vi "Test_Window.vi"() -> ()   [LabVIEW 2018]
uses:
  _TypeDefs/Flags/Z900_navX_Flags_HardwareRevTypeDef.ctl
  _TypeDefs/Flags/Z900_navX_Flags_OmnimountConfigTypeDef.ctl
  _TypeDefs/Flags/Z900_navX_Flags_OpStatusTypeDef.ctl
  _TypeDefs/Flags/Z900_navX_Flags_CalibrationStatusTypeDef.ctl
  _TypeDefs/Z900_navX_SerialStreamTypeDef.ctl
  _TypeDefs/FRIC_navX_DeviceNumbersTypeDef.ctl
panel:
  in  "Tab Control":enum32{"Device 0", "Device 1"}(tab)
  out "Warning":bool
  in  "Change Serial Stream":bool
  out "Connected":bool
  out "Displacement":T1 {"Velocity X" format="%.8f"; "Velocity Y" format="%.8f"; "Velocity Z" format="%.8f"; "Displace X" format="%.8f"; "Displace Y" format="%.8f"; "Displace Z" format="%.8f"}
  out "MPUTemp":dbl format="%.2f"
  out "Board Information":T4 {"Board"."Hardware Revision" items=["navX-MXP"=33, "navX-Micro"=40]; "Omnimount Config" items=["DEFAULT", "X_UP", "X_DOWN", "Y_UP", "Y_DOWN", "Z_UP", "Z_DOWN"]}
  out "Linear Acceleration":cluster{"X":dbl, "Y":dbl, "Z":dbl} {"X" format="%.6f"; "Y" format="%.6f"; "Z" format="%.6f"}
  out "Quaternion":T5 {"Quat W" format="%.8f"; "Quat X" format="%.8f"; "Quat Y" format="%.8f"; "Quat Z" format="%.8f"}
  out "Status":T8 {"OP Status" items=["INITIALIZING", "SELFTEST_IN_PROGRESS", "ERROR", "IMU_AUTOCAL_IN_PROGRESS", "NORMAL"]; "Calibration Status" items=["IMU_CAL_STATE_MASK"=3, "IMU_CAL_STATE_INPROGRESS"=0, "IMU_CAL_STATE_ACCUMULATE"=1, "IMU_CAL_STATE_COMPLETE"=2]}
  out "YRPHfH":T9 {"Yaw" format="%.2f"; "Roll" format="%.2f"; "Pitch" format="%.2f"; "Heading" format="%.2f"; "Fused Heading" format="%.2f"}
  out "Timestamp":u32
  out "Error":bool
  out "error":errorcluster
  in  "Zero Yaw":bool
  in  "Zero Displacement":bool
  in  "Zero Velocity":bool
  out "Raw Values":T10 {"Accel X" format="%.8f"; "Accel Y" format="%.8f"; "Accel Z" format="%.8f"; "Gyro X" format="%.8f"; "Gyro Y" format="%.8f"; "Gyro Z" format="%.8f"; "Mag X" format="%.8f"; "Mag Y" format="%.8f"; "Mag Z" format="%.8f"}
  in  "Stream Type":T11=enum."AHRSAndPositioning"
  in  "Device Number":T12
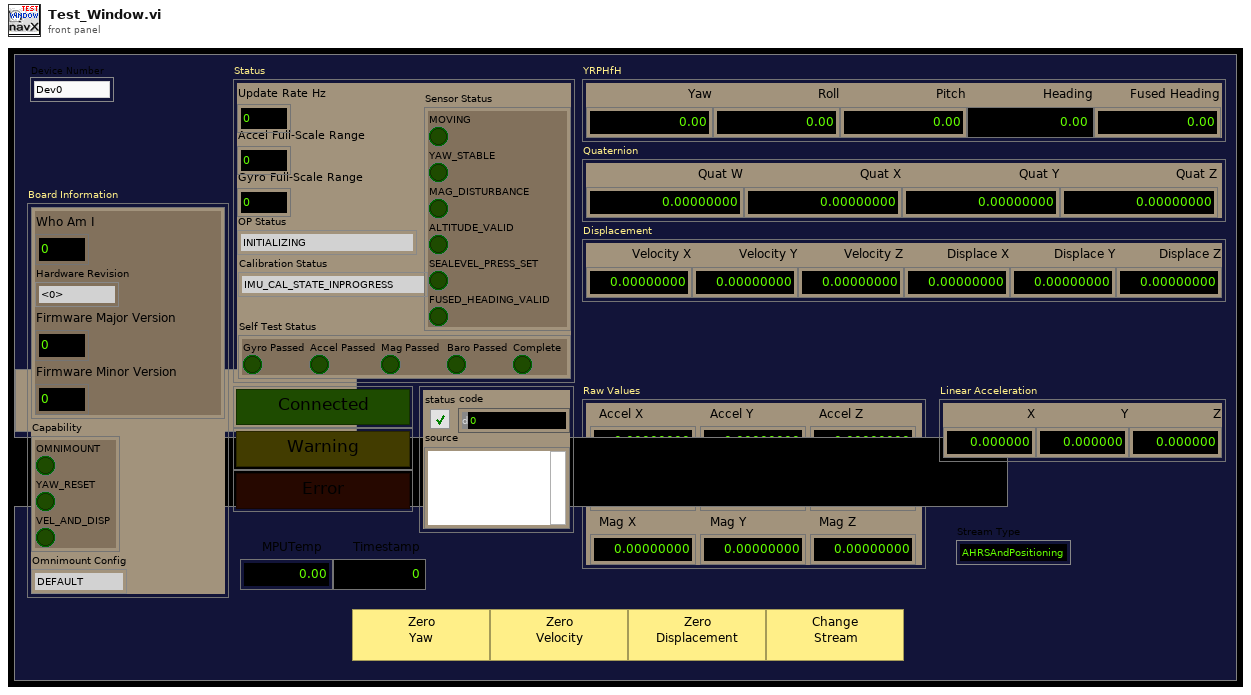
[diagram p1: front panel]
types:
  T1 = cluster{"Velocity X":dbl, "Velocity Y":dbl, "Velocity Z":dbl, "Displace X":dbl, "Displace Y":dbl, "Displace Z":dbl}
  T2 = typedef "Z900_navX_Flags_HardwareRevTypeDef.ctl" = u8
  T3 = typedef "Z900_navX_Flags_OmnimountConfigTypeDef.ctl" = u8
  T4 = cluster{"Board":cluster{"Who Am I":u8, "Hardware Revision":T2, "Firmware Major Version":u8, "Firmware Minor Version":u8}, "Capability":cluster{"OMNIMOUNT":bool, "YAW_RESET":bool, "VEL_AND_DISP":bool}, "Omnimount Config":T3}
  T5 = cluster{"Quat W":dbl, "Quat X":dbl, "Quat Y":dbl, "Quat Z":dbl}
  T6 = typedef "Z900_navX_Flags_OpStatusTypeDef.ctl" = u8
  T7 = typedef "Z900_navX_Flags_CalibrationStatusTypeDef.ctl" = u8
  T8 = cluster{"Update Rate Hz":u8, "Accel Full-Scale Range":u8, "Gyro Full-Scale Range":u16, "OP Status":T6, "Calibration Status":T7, "Sensor Status":cluster{"MOVING":bool, "YAW_STABLE":bool, "MAG_DISTURBANCE":bool, "ALTITUDE_VALID":bool, "SEALEVEL_PRESS_SET":bool, "FUSED_HEADING_VALID":bool}, "Self Test Status":cluster{"Gyro Passed":bool, "Accel Passed":bool, "Mag Passed":bool, "Baro Passed":bool, "Complete":bool}}
  T9 = cluster{"Yaw":dbl, "Roll":dbl, "Pitch":dbl, "Heading":dbl, "Fused Heading":dbl}
  T10 = cluster{"Accel X":dbl, "Accel Y":dbl, "Accel Z":dbl, "Gyro X":dbl, "Gyro Y":dbl, "Gyro Z":dbl, "Mag X":dbl, "Mag Y":dbl, "Mag Z":dbl}
  T11 = typedef "Z900_navX_SerialStreamTypeDef.ctl" = enum16{"YRPH", "Quaterinons", "Gyro/Raw", "AHRS", "AHRSAndPositioning", "AHRSAndPOSTime"}
  T12 = typedef "FRIC_navX_DeviceNumbersTypeDef.ctl" = enum16{"Dev0", "Dev1", "Dev2", "Dev3"}
  T13 = cluster{"Velocity X":dbl, "Velocity Y":dbl, "Velocity Z":dbl, "Displacement X":dbl, "Displacement Y":dbl, "Displacement Z":dbl}
  T14 = cluster{"LinearAcceleration X":dbl, "LinearAcceleration Y":dbl, "LinearAcceleration Z":dbl}
  T15 = cluster{"Update Rate Hz":u8, "Accelerometer Full-Scale Range":u8, "Gyro Full-Scale Range":u16, "OP Status":T6, "Calibration Status":T7, "Sensor Status":cluster{"MOVING":bool, "YAW_STABLE":bool, "MAG_DISTURBANCE":bool, "ALTITUDE_VALID":bool, "SEALEVEL_PRESS_SET":bool, "FUSED_HEADING_VALID":bool}, "Self Test Status":cluster{"Gyro Passed":bool, "Accel Passed":bool, "Mag Passed":bool, "Baro Passed":bool, "Complete":bool}}
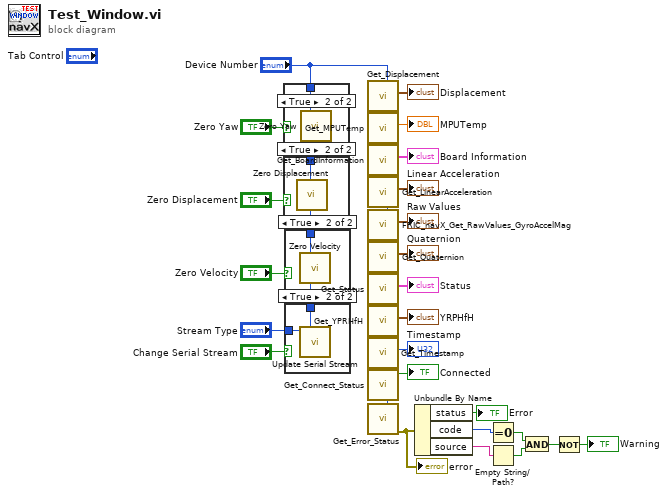
[diagram p0: block diagram]
diagram:
  n1 = case shown="True" "Zero Yaw" {
    tunnel: "Device Number" -> [_ w25]
    frame False {
    }
    frame True {
      n2 = call "Zero Yaw.vi"("Device Number"=w25) -> ()  [unwired: 11 in]
    }
  }
  n3 = case shown="True" "Zero Displacement" {
    tunnel: "Device Number" -> [_ w26]
    frame False {
    }
    frame True {
      n4 = call "Zero Displacement.vi"("Device Number"=w26) -> ()  [unwired: 11 in]
    }
  }
  n5 = case shown="True" "Zero Velocity" {
    tunnel: "Device Number" -> [_ w27]
    frame False {
    }
    frame True {
      n6 = call "Zero Velocity.vi"("Device Number"=w27) -> ()  [unwired: 11 in]
    }
  }
  n7 = case shown="True" "Change Serial Stream" {
    tunnel: "Device Number" -> [_ w29]
    tunnel: "Stream Type" -> [_ w28]
    frame False {
    }
    frame True {
      n8 = call "Update Serial Stream.vi"("Device Number"=w29, "Stream Type"=w28) -> ()  [unwired: 10 in]
    }
  }
  n9 = call "Get_Displacement.vi"("Device Number"="Device Number") -> ("Displacement"=→"Displacement":T13)  [unwired: 10 in]
  n10 = call "Get_MPUTemp.vi"("Device Number"="Device Number") -> ("MPUTemp"=→"MPUTemp":dbl)  [unwired: 10 in]
  n11 = call "Get_BoardInformation.vi"("Device Number"="Device Number") -> ("Board Information"=→"Board Information":T4)  [unwired: 10 in]
  n12 = call "Get_LinearAcceleration.vi"("Device Number"="Device Number") -> ("Linear Acceleration"=→"Linear Acceleration":T14)  [unwired: 10 in]
  n13 = call "FRIC_navX_Get_RawValues_GyroAccelMag.vi"("Device Number"="Device Number") -> ("Raw Values (out)"=→"Raw Values":T10)  [unwired: 10 in]
  n14 = call "Get_Quaternion.vi"("Device Number"="Device Number") -> ("Quaternion"=→"Quaternion":T5)  [unwired: 10 in]
  n15 = call "Get_Status.vi"("Device Number"="Device Number") -> ("Status"=→"Status":T15)  [unwired: 10 in]
  n16 = call "Get_YPRHfH.vi"("Device Number"="Device Number") -> ("YRPHfH"=→"YRPHfH":T9)  [unwired: 10 in]
  n17 = call "Get_Timestamp.vi"("Device Number"="Device Number") -> ("Timestamp"=→"Timestamp":u32)  [unwired: 10 in]
  n18 = call "Get_Connect_Status.vi"("Device Number"="Device Number") -> ("Connected"=→"Connected":bool)  [unwired: 10 in]
  n19 = call "Get_Error_Status.vi"("Device Number"="Device Number") -> ("error out"=w8:errorcluster)  [unwired: 10 in]
  "error" <- w8
  n20 = Unbundle By Name(w8) -> ("status"=→"Error":bool, "code"=w6:i32, "source"=w5:string)
  n21 = Equal To 0?(x=w6) -> (x = 0?=w4:bool)
  n22 = Empty String/Path?(string/path=w5) -> (empty?=w3:bool)
  n23 = And(x=w4, y=w3) -> (x .and. y?=w2:bool)
  n24 = Not(x=w2) -> (.not. x?=→"Warning":bool)
